vi "Get Shared Status Variable References and Descriptions.vi"(8 "error in":errorcluster) -> (0 "error out":errorcluster, 3 "Shared Variables and Descriptions":T1[](array[typedef]))   [LabVIEW 2017, in "Status Monitor Library.lvlib"]
doc: "Get references and description, for all status variables\n\n-Find all shared variables which hold status messages\n-Open a read-only connection to that shared variable\n-Return the array of relevant shared variables, with their descriptions"
uses:
  Status Monitor Library.lvlib
  Network Shared Variables/Typedefs/Share Variable and Description--Cluster.ctl
  Network Shared Variables/Typedefs/Shared Variable Properties--Cluster.ctl
  Communications/Typedefs/DTACQ Module Carrier Status.ctl
  Communications/Typedefs/DTACQ Status--Enum.ctl
  Network Shared Variables/Shared Variables Library.lvlib
  Communications/Communications Library.lvlib
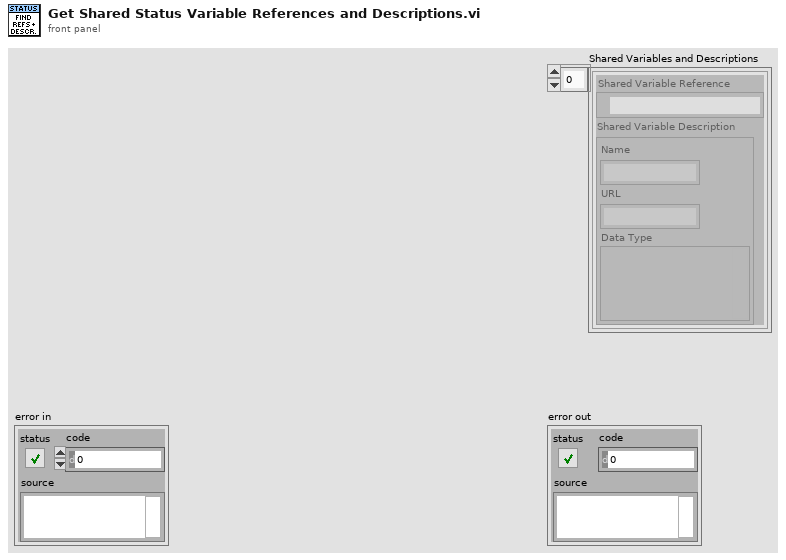
[diagram p1: front panel]
types:
  T1 = typedef "Shared Variables Library.lvlib/Share Variable and Description--Cluster.ctl" = cluster{"Shared Variable Reference":refnum<k21>, "Shared Variable Description":T2}
  T2 = typedef "Shared Variables Library.lvlib/Shared Variable Properties--Cluster.ctl" = cluster{"Name":string, "URL":string, "Data Type":variant}
  T3 = cluster{"Read Access":enum8{"Allowed", "Required", "None"}, "Write Access":enum8{"Allowed", "Required", "None"}}
  T4 = typedef "Communications Library.lvlib/DTACQ Module Carrier Status.ctl" = cluster{"DTACQ State":T5, "Pre-Trigger Samples":i32, "Post-Trigger Samples":i32, "Total Samples":i32, "Post Processing":bool}
  T5 = typedef "Communications Library.lvlib/DTACQ Status--Enum.ctl" = enum16{"IDLE", "ARM", "RUN_PRE-TRIGGER", "RUN_POST-TRIGGER", "POST_PROCESS", "CLEANUP"}
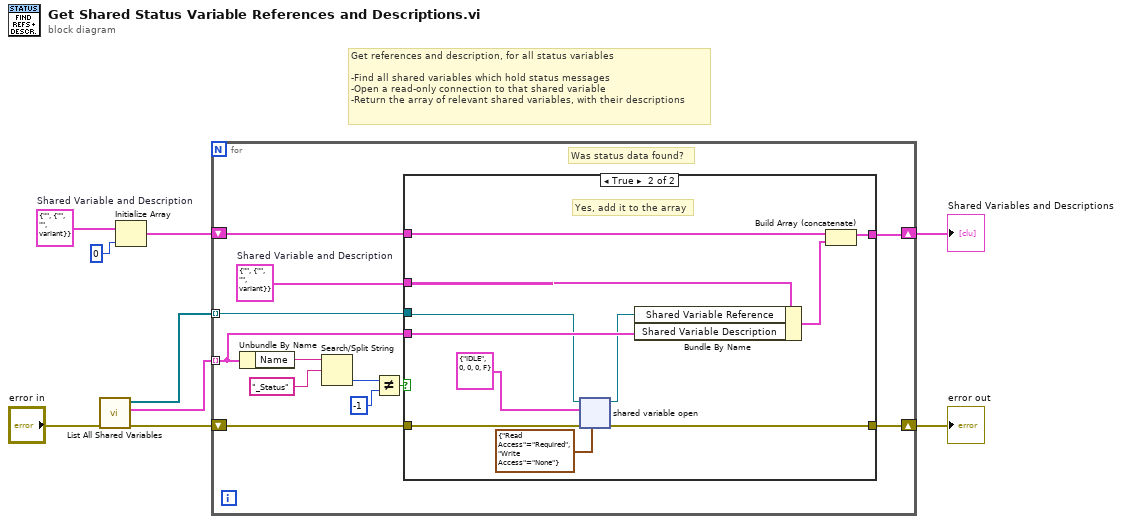
[diagram p0: block diagram]
diagram:
  w5 = T1 {"Shared Variable Reference"="", "Shared Variable Description"={"Name"="", "URL"="", "Data Type"=variant}}  # Shared Variable and Description
  # "Get references and description, for all status variables\n\n-Find all shared variables which hold status messages\n-Open a read-only connection to that shared variable\n-Return the array of relevant shared variables, with their descriptions"
  n1 = call "List All Shared Variables.vi"("error in"="error in") -> ("error out"=w7:errorcluster, "Variable Descriptions"=w2:T2[], "Variable References"=w6:refnum<k21>[])  [unwired: 8 in]
  n2 = Initialize Array(w5, 0 ("dimension size")) -> (w4:T1[])
  n3 = for {
    tunnel: w2 -> [w15] mode=indexing
    shift-right: [w14] -> w9
    shift-left: w4 -> [w17]
    tunnel: w6 -> [w12] mode=indexing
    shift-right: [w10] -> w8
    shift-left: w7 -> [w11]
    w13 = T1 {"Shared Variable Reference"="", "Shared Variable Description"={"Name"="", "URL"="", "Data Type"=variant}}  # Shared Variable and Description
    # "Was status data found?"
    n4 = Unbundle By Name(w15) -> ("Name"=w21:string)
    n5 = Search/Split String(string=w21, search string/char (-)="_Status") -> (offset of match=w19:i32)  [unwired: 1 in, 2 out]
    n6 = Not Equal?(x=w19, y=-1) -> (x != y?=w16:bool)
    n7 = case shown="True" w16 {
      tunnel: w17 -> [w23 w34]
      tunnel: w15 -> [_ w31]
      tunnel: [w23 w33] -> w14
      tunnel: w13 -> [_ w32]
      tunnel: w12 -> [_ w28]
      tunnel: w11 -> [w22 w29]
      tunnel: [w22 w24] -> w10
      frame False {
        # "No, not status data.\nDo not add to array."
      }
      frame True {
        # "Yes, add it to the array"
        n8 = shared-variable-open(w28, w29, T4 {"DTACQ State"=enum."IDLE", "Pre-Trigger Samples"=0, "Post-Trigger Samples"=0, "Total Samples"=0, "Post Processing"=FALSE} ("Module Carrier Status"), T3 {"Read Access"=enum."Required", "Write Access"=enum."None"} ("access")) -> (w27:refnum<k21>, w24:errorcluster)
        n9 = Bundle By Name(cluster=w32, "Shared Variable Reference"=w27, "Shared Variable Description"=w31) -> (w30:T1)
        n10 = Build Array (concatenate)(w34, w30) -> (w33:T1[])
      }
    }
  }
  "Shared Variables and Descriptions" <- w9
  "error out" <- w8
